vi "OpenCV.vi"() -> ()   [LabVIEW 2019]
panel:
  in  "stop":bool
  in  "Path":path
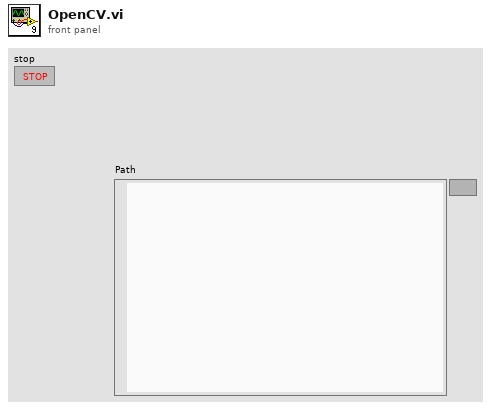
[diagram p1: front panel]
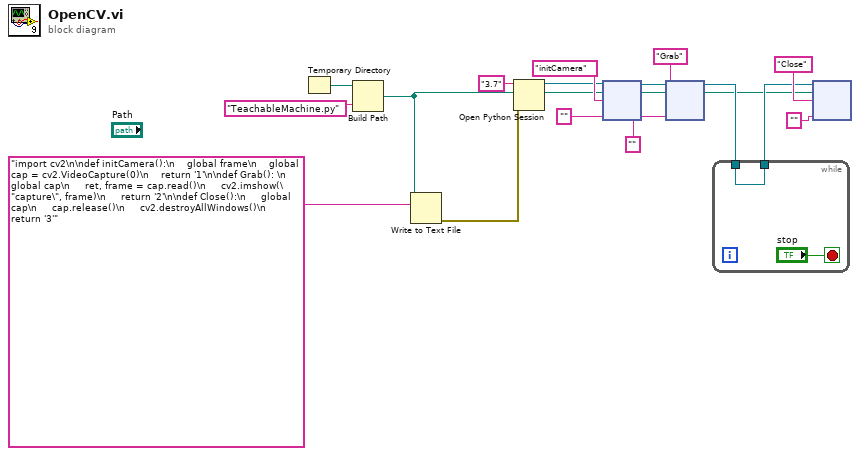
[diagram p0: block diagram]
diagram:
  n1 = Temporary Directory() -> (w15:path)
  n2 = Build Path(base path=w15, name or relative path="TeachableMachine.py") -> (appended path=w1:path)
  n3 = Write to Text File(file (use dialog)=w1, text="import cv2\n\ndef initCamera():\n    global frame\n    global cap = cv2.VideoCapture(0)\n    return '1'\n\ndef Grab(): \n     global cap\n     ret, frame = cap.read()\n     cv2.imshow(\"capture\", frame)\n     return '2'\n\ndef Close():\n     global cap\n     cap.release()\n     cv2.destroyAllWindows()\n     return '3'" ("name or relative path")) -> (error out=w8:errorcluster)  [unwired: 2 in, 2 out]
  n4 = Open Python Session(python version="3.7" ("Python version"), 3:w8) -> (session out=w12:refnum<k35>)  [unwired: 1 in, 1 out]
  n5 = node(w12, w1, "initCamera" ("function name"), "" ("function name")) -> (w6:refnum<k35>)  [unwired: 2 in, 3 out]
  n6 = node(w6, w1, "Grab" ("function name"), "" ("function name")) -> (w2:refnum<k35>)  [unwired: 2 in, 3 out]
  n7 = while {
    tunnel: [w17] -> w3
    tunnel: w2 -> [w17]
    stop <- "stop" stop-if-true
  }
  n8 = node(w3, w1, "Close" ("function name"), "" ("function name")) -> ()  [unwired: 2 in, 4 out]
